vi "AutoWriterCluster.vi"(0 "Mode(Write=True)":bool, 2 "Input":T1) -> (1 "Output":T1)   [LabVIEW 2010, in "Recorder.lvlib"]
uses:
  Recorder.lvlib
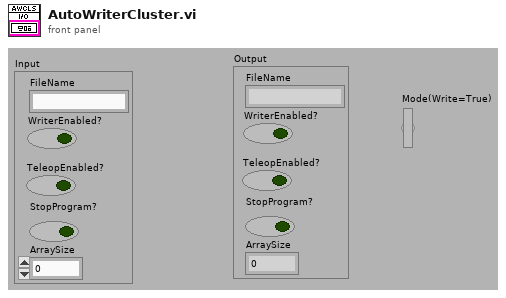
[diagram p1: front panel]
types:
  T1 = cluster{"FileName":string, "WriterEnabled?":bool, "TeleopEnabled?":bool, "StopProgram?":bool, "ArraySize":u8}
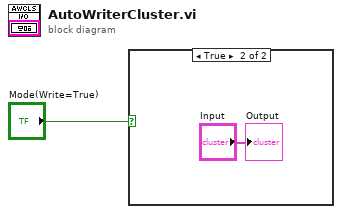
[diagram p0: block diagram]
diagram:
  n1 = case shown="True" "Mode(Write=True)" {
    frame False {
    }
    frame True {
      "Output" <- "Input"
    }
  }
